vi "DSF.Engine.Interface.Builder.Read.Command.vi"(8 "error in (no error)":errorcluster, 9 "timeout in ms (0)":i32, 11 "Builder Interface in":refnum<class "DSF.Engine.Interface.Builder.lvclass">) -> (0 "error out":errorcluster, 1 "empty?":bool, 2 "command":T1, 3 "Builder Interface out":refnum<class "DSF.Engine.Interface.Builder.lvclass">, 4 "# elements":u32)   [LabVIEW 2016, in "DSF.Engine.lvlib" / "DSF.Engine.Interface.Builder.lvclass"]
uses:
  DSF.Engine.Interface.Builder.lvclass
  C:/Git/Sourcetree/DSF/Source/Engine/Classes/Interface/DSF.Engine.Interface.lvclass
  DSF.Engine.Interface.Builder.Command Data.ctl
  DSF.Engine.Interface.Builder.Command.ctl
  DSF.Engine.Interface.lvclass/DSF.Engine.Interface.ctl
  DSF.Engine.Interface.lvclass
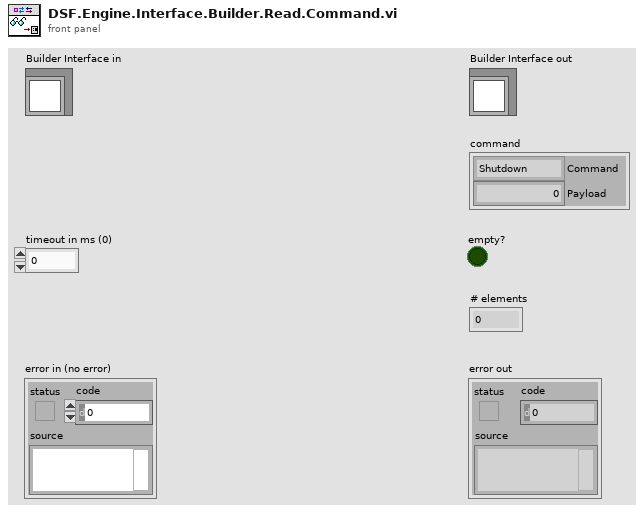
[diagram p1: front panel]
types:
  T1 = typedef "DSF.Engine.lvlib/DSF.Engine.Interface.Builder.lvclass/DSF.Engine.Interface.Builder.Command Data.ctl" = cluster{"Command":T2, "Payload":u64}
  T2 = typedef "DSF.Engine.lvlib/DSF.Engine.Interface.Builder.lvclass/DSF.Engine.Interface.Builder.Command.ctl" = enum8{"Shutdown"}
  T3 = typedef "DSF.Engine.lvlib/DSF.Engine.Interface.lvclass/DSF.Engine.Interface.RT FIFO Ref.ctl" = refnum<k33>
  T4 = typedef "DSF.Engine.lvlib/DSF.Engine.Interface.lvclass/DSF.Engine.Interface.RT FIFO Data.ctl" = cluster{"Command":u8, "Payload":u64}
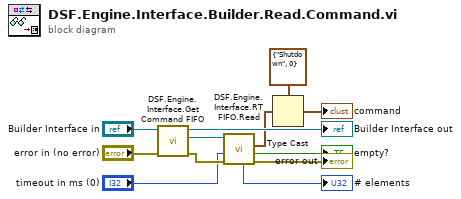
[diagram p0: block diagram]
diagram:
  n1 = call "DSF.Engine.Interface.Get Command FIFO.vi"("error in (no error)"="error in (no error)", "Interface in"="Builder Interface in") -> ("error out"=w11:errorcluster, "Command FIFO"=w12:T3, "Interface out"=→"Builder Interface out":refnum<class "DSF.Engine.Interface.Builder.lvclass">)  [unwired: 7 in]
  n2 = call "DSF.Engine.Interface.RT FIFO.Read.vi"("error in (no error)"=w11, "timeout in ms (0)"="timeout in ms (0)", "RT FIFO in"=w12) -> ("error out"=→"error out":errorcluster, "empty?"=→"empty?":bool, "element out"=w1:T4, "# elements"=→"# elements":u32)  [unwired: 4 in, 1 out]
  n3 = Type Cast(type=T1 {"Command"=enum."Shutdown", "Payload"=0} ("Plugin Command"), x=w1) -> (*(type *) &x=→"command":T1)
